vi "HD3000test.vi"() -> ()   [LabVIEW 2013]
uses:
  <vilib>/vision/NI_Vision_Development_Module.lvlib
  <vilib>/ptbypt/NI_PtbyPt.lvlib
  <vilib>/Utility/file.llb/Write To Spreadsheet File (DBL).vi
  <vilib>/Utility/file.llb/Read From Spreadsheet File (DBL).vi
panel:
  out "Mean Value":sgl
  out "Frame Rate":dbl
  in  "Display":bool=TRUE
  in  "Rec":bool
  in  "Start":bool
  in  "?":enum32{"Settings", "Monitor", "Errors"}(tab)
  in  "Selected Path for AVI":path
  in  "Auto":bool
  in  "Auto":bool
  in  "Exposure":dbl(slide)=0.00048828125 caption="Exposure::Value" min=0.00048828125 max=2.0 scale=0.00048828125..2.0 scale format="%#_1f"
  in  "White Balance":i64(slide)=3040 caption="White Balance::Value" min=2800 max=8000 step=1 scale=2800.0..10000.0
  in  "Sharpness":i64(slide)=25 caption="Sharpness::Value" min=0 max=50 step=1 scale=0.0..50.0
  in  "Saturation":i64(slide)=83 caption="Saturation::Value" min=0 max=200 step=1 scale=0.0..200.0
  in  "Contrast":dbl(slide)=0.05 caption="Contrast::Value" min=0.0 max=0.1 scale=0.0..0.1
  in  "Brightness":i64(slide)=133 caption="Brightness::Value" min=30 max=255 step=1 scale=30.0..255.0
  out "Rec Time":dbl format="%#_3g"
  out "Est. fps":dbl format="%#_2g"
  out "Frames Recorded":dbl
  out "Frames not Recorded":dbl
  out "Image Number":u32
  out "Lost Image Count":u32
  out "Total Images Transferred":u32
  in  "Interface Name":string="cam1"
  out "error out":errorcluster
  out "Histogram":T1(graph)
  out "Image":T2(plugin-control)
  in  "Stop (F)":bool
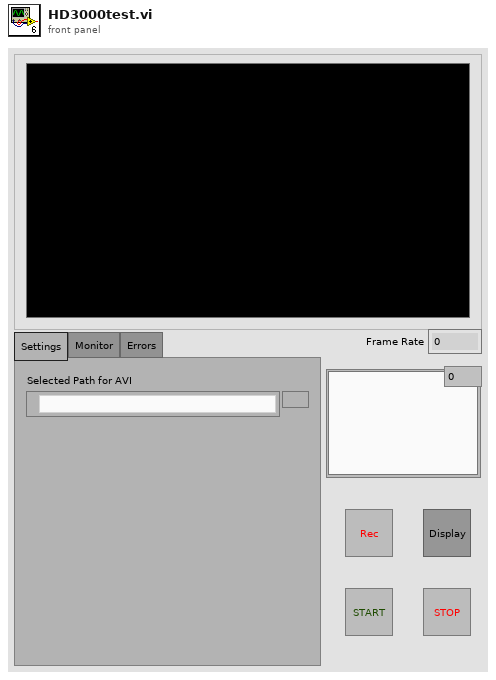
[diagram p1: front panel]
types:
  T1 = cluster{"Starting Value":sgl, "Incremental Value":sgl, "Histogram":u32[]}
  T2 = typedef "IMAQ Image.ctl" = refnum<image>
  T3 = typedef "Image Type" = u32
  T4 = typedef "AviRefnum.ctl" = refnum<k1>
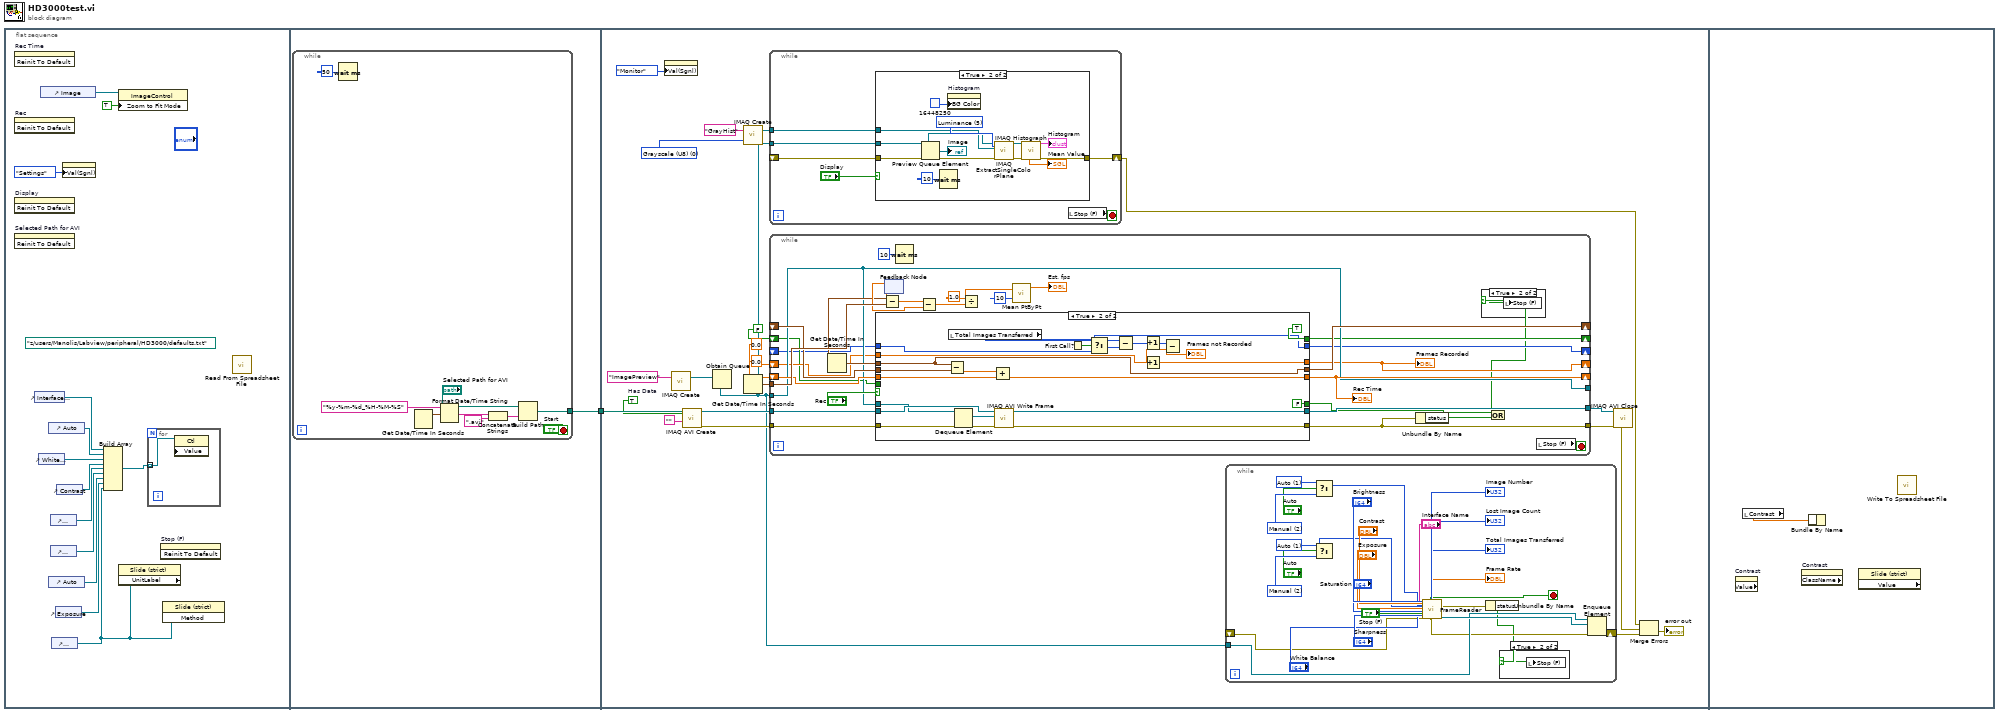
[diagram p0: block diagram]
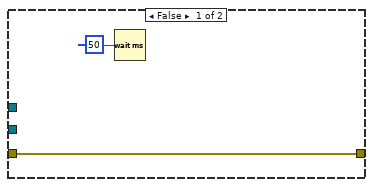
[diagram p2: hidden frame]
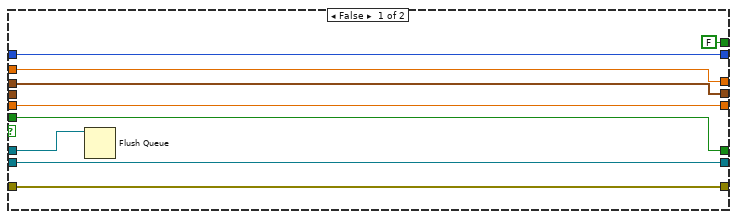
[diagram p5: hidden frame]
diagram:
  n1 = flat-sequence {
    tunnel: [w16] -> w1
    tunnel: w1 -> [w43]
    frame #0 {
      (unwired) path "z:/users/Manolis/Labview/peripheral/HD3000/defaults.txt" ("file path (dialog if empty)")
      n2 = invoke on="Rec Time" class="DigNum (strict)" method="Reinit To Default"() -> ()  [unwired: 3 in, 3 out]
      n3 = invoke on="Rec" class="Bool (strict)" method="Reinit To Default"() -> ()  [unwired: 3 in, 3 out]
      n4 = invoke on="Display" class="Bool (strict)" method="Reinit To Default"() -> ()  [unwired: 3 in, 3 out]
      n5 = invoke on="Selected Path for AVI" class="Path" method="Reinit To Default"() -> ()  [unwired: 3 in, 3 out]
      n6 = control-ref of="Interface Name"() -> (w11:refnum<vi>)
      n7 = control-ref of="White Balance"() -> (w9:refnum<vi>)
      n8 = control-ref of="Image"() -> (w12:refnum<vi>)
      n9 = control-ref of="Auto"() -> (w10:refnum<vi>)
      n10 = control-ref of="Auto"() -> (w5:refnum<vi>)
      n11 = control-ref of="Saturation"() -> (w7:refnum<vi>)
      n12 = control-ref of="Brightness"() -> (w6:refnum<vi>)
      n13 = control-ref of="Sharpness"() -> (w2:refnum<vi>)
      n14 = control-ref of="Exposure"() -> (w4:refnum<vi>)
      n15 = control-ref of="Contrast"() -> (w8:refnum<vi>)
      n16 = property class="TabCtl (strict)"("Val(Sgnl)"=enum32{"Settings", "Monitor"}."Settings" ("Value (Signaling)")) -> ()  [unwired: 2 in, 2 out]
      n17 = Build Array(w11, w10, w9, w8, w7, w6, w5, w4, w2) -> (w3:refnum<vi>[])
      n18 = property on="Property Node" class="ImageControl"(reference=w12, "Zoom to Fit Mode"=TRUE) -> ()  [unwired: 1 in, 2 out]
      n19 = property class="Slide (strict)" props=["UnitLabel"](reference=w2) -> ()  [unwired: 1 in, 3 out]
      n20 = for {
        tunnel: w3 -> [w15] mode=indexing
        n21 = property class="Ctl" props=["Value"](reference=w15) -> ()  [unwired: 2 in, 2 out]
      }
      n22 = invoke on="Stop (F)" class="Bool (strict)" method="Reinit To Default"() -> ()  [unwired: 3 in, 3 out]
      n23 = invoke class="Slide (strict)" method=#-1(reference=w2) -> ()  [unwired: 2 in, 3 out]
      n24 = call-poly <vilib>:"Read From Spreadsheet File.vi"() -> ()  [unwired: 7 in, 5 out]
    }
    frame #1 {
      n25 = while {
        tunnel: [w17] -> w16
        stop <- "Start" stop-if-true
        n26 = Wait (ms)(milliseconds to wait=u32 50) -> ()  [unwired: 1 out]
        n27 = Get Date/Time In Seconds() -> (seconds since 1Jan1904=w23:timestamp)
        n28 = Format Date/Time String(time format string (%c)="%y-%m-%d_%H-%M-%S", seconds (now)=w23) -> (date/time string=w21:string)  [unwired: 1 in]
        n29 = Concatenate Strings(w21, ".avi" ("search string")) -> (w19:string)
        n30 = Build Path(base path="Selected Path for AVI", name or relative path=w19) -> (appended path=w17:path)
      }
    }
    frame #2 {
      w37 = T3 0 items=["Grayscale (U8)", "Grayscale (I16)", "Grayscale (SGL)", "Complex (CSG)", "RGB (U32)", "HSL (U32)", "RGB (U64)", "Grayscale (U16)"] ("Image Type")
      w39 = TRUE  # Has Data
      n31 = property class="TabCtl (strict)"("Val(Sgnl)"=enum32{"Settings", "Monitor"}."Monitor" ("Value (Signaling)")) -> ()  [unwired: 2 in, 2 out]
      n32 = call "IMAQ Create"("Image Name"="ImagePreview") -> ("New Image"=w33:T2)  [unwired: 4 in, 1 out]
      n33 = call "IMAQ AVI Create"("Has Data"=w39, "Compression Filter"="", "AVI Path"=w43) -> ("error out"=w44:errorcluster, "Avi Refnum"=w47:T4)  [unwired: 4 in, 3 out]
      n34 = Obtain Queue(element data type=w33) -> (queue out=w32:refnum<queue>)  [unwired: 4 in, 2 out]
      n35 = call "IMAQ Create"("Image Name"="GrayHist", "Image Type"=w37) -> ("New Image"=w35:T2)  [unwired: 3 in, 1 out]
      n36 = Get Date/Time In Seconds() -> (seconds since 1Jan1904=w41:timestamp)
      n37 = while {
        tunnel: w32 -> [w51]
        tunnel: w35 -> [w52]
        shift-right: [w49] -> w26
        shift-left: _ -> [w48]
        stop <- w53 stop-if-true
        n38 = case shown="True" "Display" {
          tunnel: w52 -> [_ w64]
          tunnel: w51 -> [_ w62]
          tunnel: [w54 w59] -> w49
          tunnel: w48 -> [w54 w58]
          frame False {
            n39 = Wait (ms)(milliseconds to wait=u32 50) -> ()  [unwired: 1 out]
          }
          frame True {
            w67 = 5 items=["Red", "Green", "Blue", "Hue", "Saturation", "Luminance", "Value", "Intensity"] ("Color Plane")
            n40 = Preview Queue Element(queue=w62, error in (no error)=w58) -> (element=w61:T2, error out=w57:errorcluster)  [unwired: 1 in, 2 out]
            "Image" <- w61
            n41 = Wait (ms)(milliseconds to wait=u32 10) -> ()  [unwired: 1 out]
            n42 = property on="Histogram" class="WFGraph (strict)"("BG Color"=u32 16448250) -> ()  [unwired: 2 in, 2 out]
            n43 = call "IMAQ ExtractSingleColorPlane"("Color Plane"=w67, "error in (no error)"=w57, "Image Dst"=w64, "Image Src"=w61) -> ("error out"=w60:errorcluster, "Image Dst Out"=w66:T2)  [unwired: 6 in]
            n44 = call "IMAQ Histograph"("error in (no error)"=w60, "Image"=w66) -> ("error out"=w59:errorcluster, "Mean Value"=→"Mean Value":sgl, "Histogram Graph"=→"Histogram":T1)  [unwired: 6 in, 1 out]
          }
        }
        n45 = local read "Stop (F)"() -> (w53:bool)
      }
      n46 = while {
        tunnel: [w126] -> w46
        tunnel: [w105] -> w45
        tunnel: w47 -> [w125]
        tunnel: w44 -> [w124]
        tunnel: w41 -> [w123]
        shift-right: [w122] -> _
        shift-left: _ -> [w121]
        shift-right: [w119] -> _
        shift-left: 0.0 -> [w120]
        tunnel: [w108] -> _
        tunnel: w32 -> [w108]
        shift-right: [w107] -> _
        shift-left: 0.0 -> [w106]
        shift-right: [w104] -> _
        shift-left: FALSE ("First Call?: T/F") -> [w103]
        shift-right: [w100] -> _
        shift-left: _ -> [w99]
        stop <- w109 stop-if-true
        n47 = Get Date/Time In Seconds() -> (seconds since 1Jan1904=w113:timestamp)
        n48 = case shown="True" "Rec" {
          tunnel: [w135 w159] -> w126
          tunnel: [w136 w158] -> w105
          tunnel: w125 -> [w135 w157]
          tunnel: w124 -> [w136 w148]
          tunnel: [w133 w152] -> w119
          tunnel: [w134 w155] -> w122
          tunnel: w113 -> [w134 w155]
          tunnel: w121 -> [_ w154]
          tunnel: w120 -> [w133 w153]
          tunnel: w108 -> [w132 w151]
          tunnel: [w131 w138] -> w107
          tunnel: w106 -> [w131 w149]
          tunnel: [FALSE ("First Call?: T/F") TRUE ("First Call?: T/F")] -> w104
          tunnel: w103 -> [w130 _]
          tunnel: [w130 FALSE ("First Call?: T/F")] -> w102
          tunnel: [w128 w142] -> w100
          tunnel: w99 -> [w128 w143]
          frame False {
            n49 = Flush Queue(queue=w132) -> ()  [unwired: 1 in, 3 out]
          }
          frame True {
            n50 = Subtract(x=w155, y=w154) -> (x-y=w156:dbl)
            n51 = local read "Total Images Transferred"() -> (w141:u32)
            n52 = Dequeue Element(queue=w151, error in (no error)=w148) -> (element=w150:T2, error out=w147:errorcluster)  [unwired: 1 in, 2 out]
            n53 = Add(x=w156, y=w153) -> (x+y=w152:dbl)
            n54 = call "IMAQ AVI Write Frame"("error in (no error)"=w147, "Image"=w150, "Avi Refnum"=w157) -> ("error out"=w158:errorcluster, "Avi Refnum (duplicate)"=w159:T4)  [unwired: 7 in]
            n55 = First Call?() -> (First Call?: T/F=w144:bool)
            n56 = Select(t=w141, s=w144, f=w143) -> (s? t:f=w142:u32)
            n57 = Subtract(x=w141, y=w142) -> (x-y=w140:u32)
            n58 = Increment(x=w140) -> (x+1=w139:u32)
            n59 = Increment(x=w149) -> (x+1=w138:dbl)
            n60 = Subtract(x=w139, y=w138) -> (x-y=→"Frames not Recorded":dbl)
          }
        }
        "Rec Time" <- w119
        "Frames Recorded" <- w107
        n61 = Subtract(x=w113, y=w123) -> (x-y=w114:dbl)
        n62 = feedback #1() -> (w118:dbl)  [unwired: 1 in]
        n63 = feedback-in #1(w114) -> ()
        n64 = Wait (ms)(milliseconds to wait=u32 10) -> ()  [unwired: 1 out]
        n65 = Subtract(x=w114, y=w118) -> (x-y=w116:dbl)
        n66 = Divide(x=1.0, y=w116) -> (x/y=w115:dbl)
        n67 = call <vilib>:"Mean PtByPt.vi"("x"=w115, "sample length"=10) -> ("mean"=→"Est. fps":dbl)  [unwired: 2 in, 1 out]
        n68 = Unbundle By Name(w105) -> ("status"=w101:bool)
        n69 = Or(x=w102, y=w101) -> (x .or. y?=w98:bool)
        n70 = case shown="True" w98 {
          selector: w98 -> [_ w127]
          frame False {
          }
          frame True {
            n71 = local write "Stop (F)"(w127) -> ()
          }
        }
        n72 = local read "Stop (F)"() -> (w109:bool)
      }
      n73 = while {
        tunnel: w32 -> [w83]
        shift-right: [w72] -> w29
        shift-left: _ -> [w74]
        stop <- w70 stop-if-true
        w76 = u32 2 items=["Auto"=1, "Manual"=2] ("Exposure::Mode")
        w77 = u32 1 items=["Auto"=1, "Manual"=2] ("Exposure::Mode")
        w81 = u32 2 items=["Auto"=1, "Manual"=2] ("Exposure::Mode")
        w82 = u32 1 items=["Auto"=1, "Manual"=2] ("Exposure::Mode")
        n74 = Select(t=w77, s="Auto", f=w76) -> (s? t:f=w78:u32)
        n75 = Select(t=w82, s="Auto", f=w81) -> (s? t:f=w79:u32)
        n76 = call "FrameReader.vi"("Brightness::Value"="Brightness", "Contrast::Value"="Contrast", "Exposure::Mode"=w79, "Exposure::Value"="Exposure", "Saturation::Value"="Saturation", "Stop (F)"="Stop (F)", "Sharpness::Value"="Sharpness", "error in"=w74, "White Balance::Mode"=w78, "White Balance::Value"="White Balance", "Interface Name"="Interface Name") -> ("Image Out"=w84:T2, "Image Number"=→"Image Number":u32, "Lost Image Count"=→"Lost Image Count":u32, "Total Images Transferred"=→"Total Images Transferred":u32, "Frame Rate"=→"Frame Rate":dbl, "Stopped"=w70:bool, "error out"=w73:errorcluster)  [unwired: 3 in, 7 out]
        n77 = Unbundle By Name(w73) -> ("status"=w71:bool)
        n78 = case shown="True" w71 {
          selector: w71 -> [_ w96]
          frame False {
          }
          frame True {
            n79 = local write "Stop (F)"(w96) -> ()
          }
        }
        n80 = Enqueue Element(queue=w83, element=w84, error in (no error)=w73) -> (error out=w72:errorcluster)  [unwired: 1 in, 2 out]
      }
      n81 = call "IMAQ AVI Close"("error in (no error)"=w45, "Avi Refnum"=w46) -> ("error out"=w30:errorcluster)  [unwired: 9 in]
      n82 = Merge Errors(w26, w30, w29) -> (→"error out":errorcluster)
    }
    frame #3 {
      n83 = property on="Contrast" class="Slide (strict)" props=["Value"]() -> ()  [unwired: 2 in, 3 out]
      n84 = local read "Contrast"() -> (w160:dbl)
      n85 = property on="Contrast" class="Slide (strict)" props=["ClassName"]() -> ()  [unwired: 2 in, 3 out]
      n86 = Bundle By Name(w160) -> ()  [unwired: 1 in, 1 out]
      n87 = property class="Slide (strict)" props=["Value"]() -> ()  [unwired: 2 in, 3 out]
      n88 = call-poly <vilib>:"Write To Spreadsheet File.vi"() -> ("file path (dialog if empty)"=w161:path)  [unwired: 7 in, 1 out]
    }
  }
